vi "Hotkeys (SubVI).vi"(6 "Iteration Quantity":dbl=0.1, 9 "Decrease":string="Turning Decrease", 10 "Increase":string="Turning Increase", 11 "Reference":refnum<vi>) -> ()   [LabVIEW 2018]
uses:
  <vilib>/Rock Robotics/Network Tables/NT Read Boolean.vi
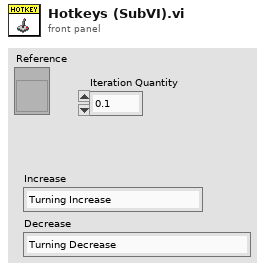
[diagram p1: front panel]
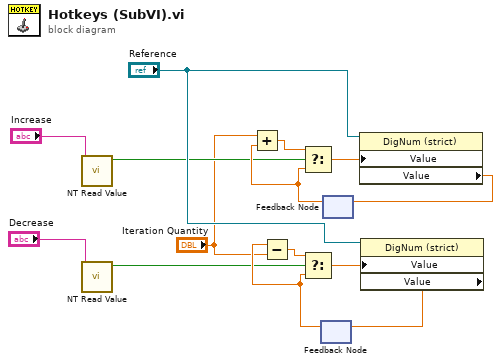
[diagram p0: block diagram]
diagram:
  n1 = call-poly <vilib>:"NT Read Value.vi"("Name"="Increase") -> ("Boolean"=w5:bool)  [unwired: 9 in, 1 out]
  n2 = call-poly <vilib>:"NT Read Value.vi"("Name"="Decrease") -> ("Boolean"=w4:bool)  [unwired: 9 in, 1 out]
  n3 = feedback #1() -> (w7:dbl)  [unwired: 1 in]
  n4 = Subtract(x=w7, y="Iteration Quantity") -> (x-y=w6:dbl)
  n5 = Select(t=w6, s=w4, f=w7) -> (s? t:f=w12:dbl)
  n6 = feedback #2() -> (w9:dbl)  [unwired: 1 in]
  n7 = Add(x="Iteration Quantity", y=w9) -> (x+y=w8:dbl)
  n8 = Select(t=w8, s=w5, f=w9) -> (s? t:f=w10:dbl)
  n9 = property class="DigNum (strict)"(reference="Reference", "Value"=w10) -> ("Value"=w11:dbl)  [unwired: 1 in, 2 out]
  n10 = feedback-in #2(w11) -> ()
  n11 = property class="DigNum (strict)"(reference="Reference", "Value"=w12) -> ("Value"=w13:dbl)  [unwired: 1 in, 2 out]
  n12 = feedback-in #1(w13) -> ()
